vi "setVXM.vi"(7 "Sub-syst number":i32, 8 "error in (no error)":errorcluster, 10 "VXMn":refnum<class "VXMx2.lvclass">, 11 "sub-systems in":refnum<class "sub-systems.lvclass">) -> (0 "error out":errorcluster, 3 "sub-systems out":refnum<class "sub-systems.lvclass">)   [LabVIEW 2018, in "sub-systems.lvclass"]
doc: "re-bundle the VXM object"
uses:
  sub-systems.lvclass
  VSMx2/VXMx2.lvclass
  sub-systems.lvclass/sub-systems.ctl
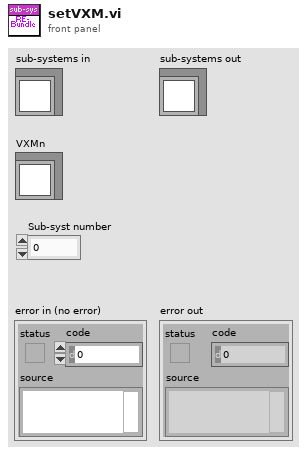
[diagram p1: front panel]
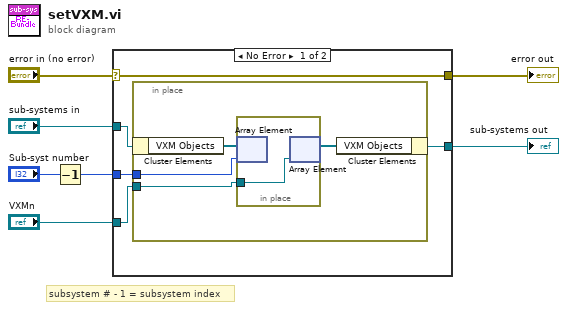
[diagram p0: block diagram]
diagram:
  # "subsystem # - 1 = subsystem index"
  n1 = Decrement(x="Sub-syst number") -> (x-1=w1:i32)
  n2 = case shown="No Error" "error in (no error)" {
    selector: "error in (no error)" -> [w12 w19]
    tunnel: [w12 w19] -> w6
    tunnel: [w10 w18] -> w4
    tunnel: "sub-systems in" -> [w11 w18]
    tunnel: w1 -> [w9 _]
    tunnel: "VXMn" -> [w8 _]
    frame No Error {
      n3 = in-place {
        in-place-border: w9 -> [w16]
        in-place-border: w8 -> [w14]
        n4 = in-place-cluster #1(w11) -> ("VXM Objects"=w15:refnum<class "VXMx2.lvclass">[])
        n5 = in-place {
          in-place-border: w14 -> [w17]
          n6 = in-place-array #2(w15, w16) -> ()  [unwired: 1 out]
          n7 = in-place-array #2(w17) -> (w13:refnum<class "VXMx2.lvclass">[])  [unwired: 1 out]
        }
        n8 = in-place-cluster #1("VXM Objects"=w13) -> (w10:refnum<class "sub-systems.lvclass">)
      }
    }
    frame Error {
    }
  }
  "error out" <- w6
  "sub-systems out" <- w4
